vi "writeToXML.vi"(8 "error in (no error)":errorcluster, 10 "ClassLabel":string, 11 "AOSPointingOffset in":refnum<class "AOSPointingOffset.lvclass">) -> (0 "error out":errorcluster, 2 "XML out":string, 3 "AOSPointingOffset out":refnum<class "AOSPointingOffset.lvclass">)   [LabVIEW 2022 SP3, in "TCSDataDefinitions.lvlib" / "TCSActiveOpticsCommand.lvlib" / "AOSPointingOffset.lvclass"]
uses:
  AOSPointingOffset.lvclass
  <userlib>/Common/UnitsAndXML/FlattenItemWithUnitToXML/FlattenPlaneAngleToXML/PlaneAngleUnit.ctl
  AOSPointingOffset.lvclass/AOSPointingOffset.ctl
  TCSActiveOpticsCommand/TCSActiveOpticsCommand.lvclass
  <userlib>/Common/UnitsAndXML/UnitsAndXML.lvlib
  <userlib>/Common/XML/XMLGenerator/XMLGenerator.lvclass
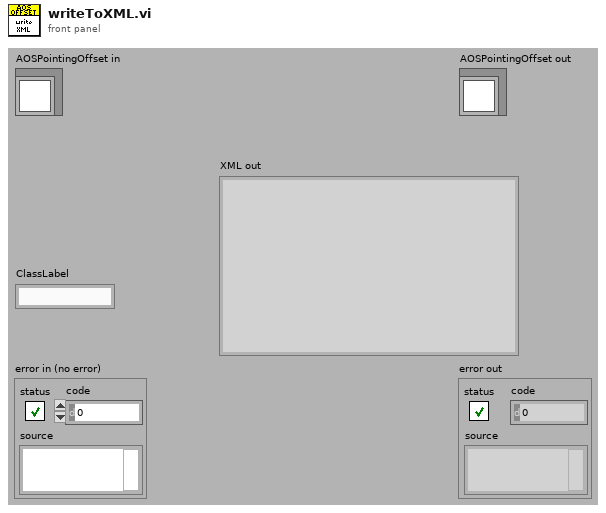
[diagram p1: front panel]
types:
  T1 = typedef "UnitsAndXML.lvlib/PlaneAngleUnit.ctl" = enum16{"rad", "deg", "'", "\""}
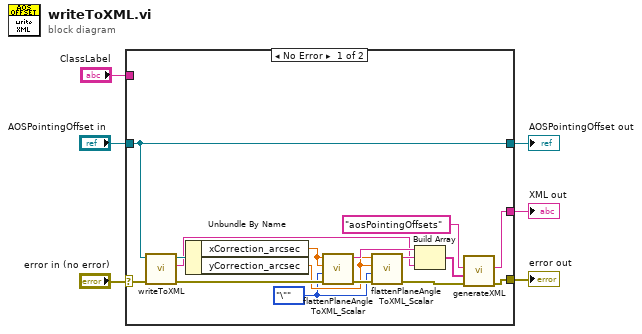
[diagram p0: block diagram]
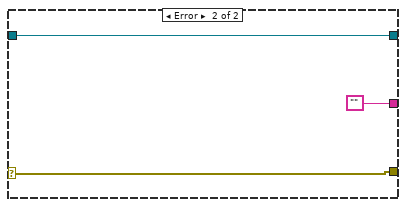
[diagram p2: hidden frame]
diagram:
  n1 = case shown="No Error" "error in (no error)" {
    selector: "error in (no error)" -> [w18 w25]
    tunnel: [w11 w25] -> w5
    tunnel: [w22 w24] -> w3
    tunnel: "AOSPointingOffset in" -> [w22 w24]
    tunnel: "ClassLabel" -> [_ _]
    tunnel: [w7 ""] -> w1
    frame No Error {
      w13 = PlaneAngleUnit."\"" ("planeAngleUnitInXML")
      n2 = call-parent "writeToXML.vi"("error in (no error)"=w18, "TCSActiveOpticsCommand in"=w22) -> ("error out"=w19:errorcluster, "XML out"=w8:string, "TCSActiveOpticsCommand out"=w21:refnum<class "AOSPointingOffset.lvclass">)  [unwired: 7 in]
      n3 = Unbundle By Name(w21) -> ("xCorrection_arcsec"=w20:dbl[unit], "yCorrection_arcsec"=w14:dbl[unit])
      n4 = call <userlib>:"flattenPlaneAngleToXML_Scalar.vi"("error in (no error)"=w19, "planeAngleUnitInXML"=w13, "planeAngleAgain"=w20, "planeAngle"=w20) -> ("error out"=w17:errorcluster, "xmlString"=w16:string)  [unwired: 6 in]
      n5 = call <userlib>:"flattenPlaneAngleToXML_Scalar.vi"("error in (no error)"=w17, "planeAngleUnitInXML"=w13, "planeAngleAgain"=w14, "planeAngle"=w14) -> ("error out"=w12:errorcluster, "xmlString"=w15:string)  [unwired: 6 in]
      n6 = Build Array(w16, w15, w8) -> (w10:string[])
      n7 = call <userlib>:"generateXML.vi"("error in"=w12, "childrenXML"=w10, "elementName"="aosPointingOffsets" ("Class Label")) -> ("error out"=w11:errorcluster, "XML out"=w7:string)  [unwired: 6 in, 1 out]
    }
    frame Error {
    }
  }
  "error out" <- w5
  "AOSPointingOffset out" <- w3
  "XML out" <- w1
